vi "GetBuvStatus (SubVI).vi"(0 "connection ID in":refnum<k5>, 5 "error in":errorcluster) -> (9 "status cluster":cluster{bool, bool, bool}, 14 "connection ID out":refnum<k5>, 16 "I Ready":bool, 19 "error out":errorcluster)   [LabVIEW 2013]
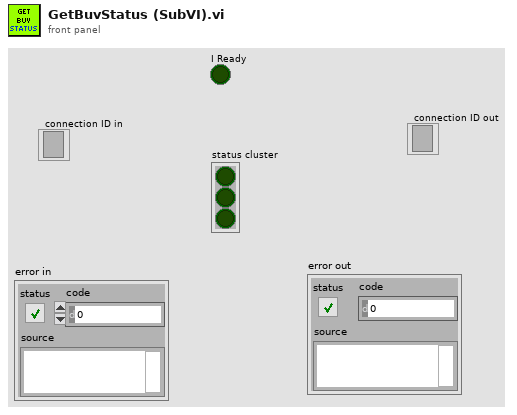
[diagram p1: front panel]
types:
  T1 = enum16{"Standard", "Buffered", "CRLF", "Immediate"}
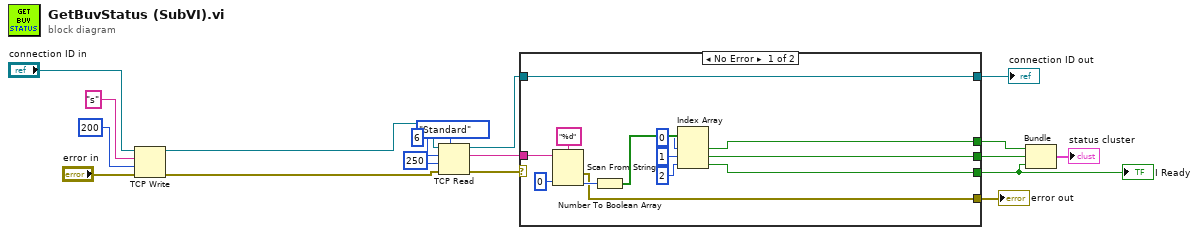
[diagram p0: block diagram]
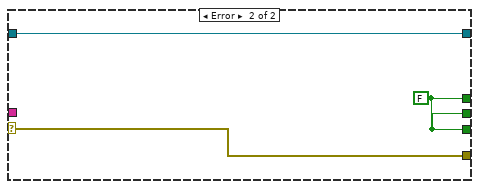
[diagram p2: hidden frame]
diagram:
  n1 = TCP Write(connection ID="connection ID in", data in="s", error in (no error)="error in", 9:200 ("timeout ms (25000)")) -> (connection ID out=w2:refnum<k5>, error out=w1:errorcluster)  [unwired: 1 out]
  n2 = TCP Read(connection ID=w2, bytes to read=6, error in (no error)=w1, 7:T1."Standard" ("mode (standard)"), 9:250 ("timeout ms (25000)")) -> (connection ID out=w18:refnum<k5>, data out=w17:string, error out=w7:errorcluster)
  n3 = case shown="No Error" w7 {
    selector: w7 -> [_ w34]
    tunnel: w17 -> [w19 _]
    tunnel: [w23 w34] -> w16
    tunnel: [w29 w33] -> w15
    tunnel: w18 -> [w29 w33]
    tunnel: [w22 w32] -> w6
    tunnel: [w21 w32] -> w5
    tunnel: [w20 w32] -> w4
    frame No Error {
      n4 = Scan From String(format string="%d", input string=w19, default 1=u8 0 ("default value 1")) -> (error out=w23:errorcluster, output 1=w28:u8)  [unwired: 2 in, 2 out]
      n5 = Number To Boolean Array(number=w28) -> (Boolean array=w27:bool[])
      n6 = Index Array(array=w27, index #1=0 ("index"), index #2=1 ("index"), index #3=2 ("index")) -> (element #1=w22:bool, element #2=w21:bool, element #3=w20:bool)
    }
    frame Error {
      w32 = FALSE
    }
  }
  "error out" <- w16
  "connection ID out" <- w15
  "I Ready" <- w4
  n7 = Bundle(w6, w5, w4) -> (→"status cluster":cluster{bool, bool, bool})  [unwired: 1 in]
